vi "Port Write (SubVI).vi"(3 "error in":errorcluster, 4 "write buffer":string, 5 "VISA Refnum in":refnum<visa-resource-name>) -> (0 "error out":errorcluster, 2 "VISA Refnum out":refnum<visa-resource-name>)   [LabVIEW 2017]
doc: "by Tanguy BOULARD"
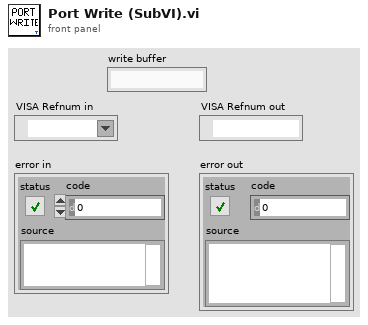
[diagram p1: front panel]
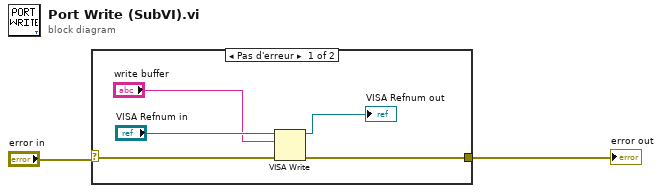
[diagram p0: block diagram]
diagram:
  n1 = case shown="Pas d'erreur" "error in" {
    selector: "error in" -> [w6 w8]
    tunnel: [w7 w8] -> w2
    frame No Error {
      n2 = VISA Write(VISA resource name="VISA Refnum in", write buffer="write buffer", error in (no error)=w6) -> (VISA resource name out=→"VISA Refnum out":refnum<visa-resource-name>, error out=w7:errorcluster)  [unwired: 1 out]
    }
    frame Error {
    }
  }
  "error out" <- w2
